vi "Scale to Fit.vi"(8 "error in (no error)":errorcluster, 9 "Actual Transform In":T1, 11 "Plot Object In":refnum<vi>) -> (0 "error out":errorcluster, 1 "Actual Transform Out":T1, 3 "Plot Object Out":refnum<vi>)   [LabVIEW 2020, in "3D Plot.lvclass"]
uses:
  3D Plot.lvclass
  Actual Transform.ctl
  Range Clusters.ctl
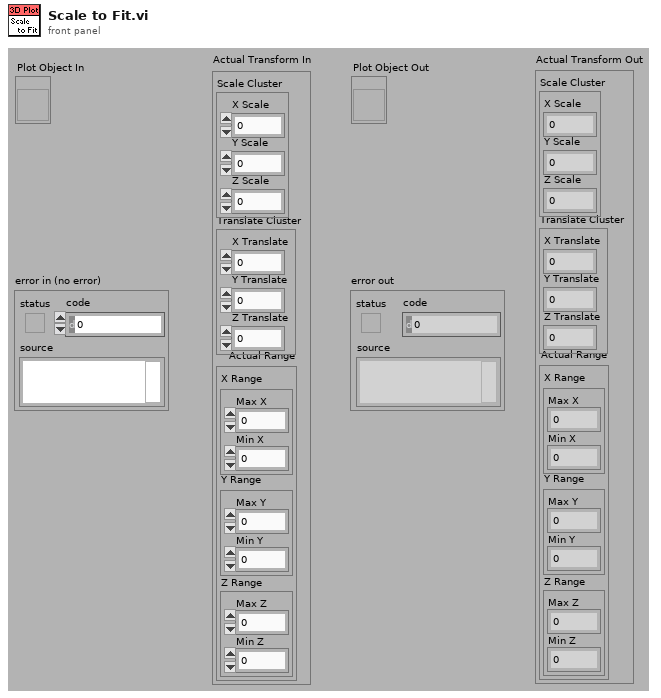
[diagram p1: front panel]
types:
  T1 = typedef "3D Plot.lvclass/Actual Transform.ctl" = cluster{"Scale Cluster":cluster{"X Scale":sgl, "Y Scale":sgl, "Z Scale":sgl}, "Translate Cluster":cluster{"X Translate":sgl, "Y Translate":sgl, "Z Translate":sgl}, "Actual Range":T2}
  T2 = typedef "3D Plot.lvclass/Range Clusters.ctl" = cluster{"X Range":cluster{"Max X":sgl, "Min X":sgl}, "Y Range":cluster{"Max Y":sgl, "Min Y":sgl}, "Z Range":cluster{"Max Z":sgl, "Min Z":sgl}}
  T3 = cluster{"X Translate":sgl, "Y Translate":sgl, "Z Translate":sgl}
  T4 = cluster{"X Scale":sgl, "Y Scale":sgl, "Z Scale":sgl}
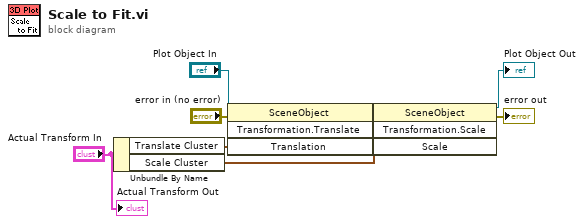
[diagram p0: block diagram]
diagram:
  n1 = Unbundle By Name("Actual Transform In") -> ("Translate Cluster"=w3:T3, "Scale Cluster"=w2:T4)
  n2 = invoke class="SceneObject" method="Transformation.Translate"(reference="Plot Object In", error in="error in (no error)", "Translation"=w3) -> (reference out=w8:refnum<vi>, error out=w5:errorcluster)  [unwired: 1 in, 2 out]
  n3 = invoke class="SceneObject" method="Transformation.Scale"(reference=w8, error in=w5, "Scale"=w2) -> (reference out=→"Plot Object Out":refnum<vi>, error out=→"error out":errorcluster)  [unwired: 1 in, 2 out]
  "Actual Transform Out" <- "Actual Transform In"
